vi "Shoot Balls.vi"(8 "error in (no error)":errorcluster, 10 "milliseconds to shoot":u32=10000) -> (0 "error out":errorcluster)   [LabVIEW 2016]
uses:
  Robot Global Data.vi
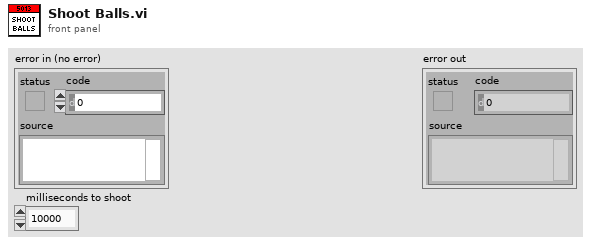
[diagram p1: front panel]
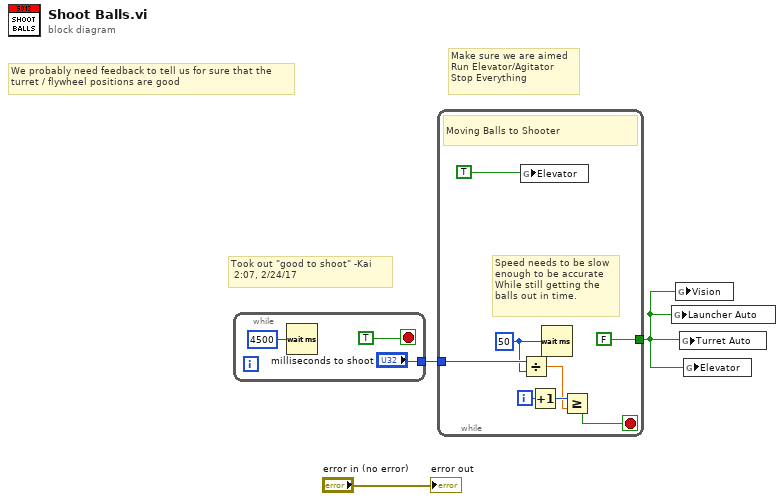
[diagram p0: block diagram]
diagram:
  # "Took out \"good to shoot\" -Kai\n 2:07, 2/24/17"
  # "We probably need feedback to tell us for sure that the\nturret / flywheel positions are good"
  # "Make sure we are aimed\nRun Elevator/Agitator\nStop Everything"
  n1 = while {
    tunnel: ["milliseconds to shoot"] -> w2
    stop <- TRUE stop-if-true
    n2 = Wait (ms)(milliseconds to wait=u32 4500) -> ()  [unwired: 1 out]
  }
  n3 = while {
    tunnel: w2 -> [w11]
    tunnel: [FALSE ("Launcher Auto")] -> w1
    i -> [w13]
    stop <- w14 stop-if-true
    w10 = u32 50 ("milliseconds to wait")
    # "Speed needs to be slow\nenough to be accurate\nWhile still getting the\nballs out in time."
    # "Moving Balls to Shooter"
    n4 = global write "Robot Global Data.vi" "Elevator"(TRUE) -> ()
    n5 = Divide(x=w11, y=w10) -> (x/y=w9:dbl)
    n6 = Increment(x=w13) -> (x+1=w12:i32)
    n7 = Wait (ms)(milliseconds to wait=w10) -> ()  [unwired: 1 out]
    n8 = Greater Or Equal?(x=w12, y=w9) -> (x >= y?=w14:bool)
  }
  n9 = global write "Robot Global Data.vi" "Launcher Auto"(w1) -> ()
  n10 = global write "Robot Global Data.vi" "Vision"(w1) -> ()
  n11 = global write "Robot Global Data.vi" "Turret Auto"(w1) -> ()
  n12 = global write "Robot Global Data.vi" "Elevator"(w1) -> ()
  "error out" <- "error in (no error)"
